vi "Graph_State_v00.vi"(4 "BS Hold Pulse":bool, 6 "\"I too high?\"":T6, 11 "Control Cavity Cluster":T11={"Control Pump A"={"Lock"=FALSE, "Hold"=FALSE, "P Gain"=0, "P BS"=-5, "I Gain"=0, "I BS"=-10, "I2 G"=0, "I2 BS"=-26, "Scan Amp"=0, "Scan Off"=0, "Scan FS"=0, "SFS BS"=0, "I Max value"=10000, "I2 Max value"=10000, "Scope.Offset"=0, "Trigger Direction"=enum."either", "Scan-PII thresh"=0}, "Control Pump B"={"Lock"=FALSE, "Hold"=FALSE, "P Gain"=0, "P BS"=-5, "I Gain"=0, "I BS"=-10, "I2 G"=0, "I2 BS"=-26, "Scan Amp"=0, "Scan Off"=0, "Scan FS"=0, "SFS BS"=0, "I Max value"=10000, "I2 Max value"=10000, "Scope.Offset"=0, "Trigger Direction"=enum."either", "Scan-PII thresh"=0}, "Control EPR"={"Lock"=FALSE, "Hold"=FALSE, "P Gain"=0, "P BS"=-5, "I Gain"=0, "I BS"=-10, "I2 G"=0, "I2 BS"=-26, "Scan Amp"=0, "Scan Off"=0, "Scan FS"=0, "SFS BS"=0, "I Max value"=10000, "I2 Max value"=10000, "Scope.Offset"=0, "Trigger Direction"=enum."either", "Scan-PII thresh"=0}, "Control Graph"={"Lock"=FALSE, "Hold"=FALSE, "P Gain"=0, "P BS"=-5, "I Gain"=0, "I BS"=-10, "I2 G"=0, "I2 BS"=-26, "Scan Amp"=0, "Scan Off"=0, "Scan FS"=0, "SFS BS"=0, "I Max value"=10000, "I2 Max value"=10000, "Scope.Offset"=0, "Trigger Direction"=enum."either", "Scan-PII thresh"=0}, "Control HD A"={"Lock"=FALSE, "Hold"=FALSE, "P Gain"=0, "P BS"=-5, "I Gain"=0, "I BS"=-10, "I2 G"=0, "I2 BS"=-26, "Scan Amp"=0, "Scan Off"=0, "Scan FS"=0, "SFS BS"=0, "I Max value"=10000, "I2 Max value"=10000, "Scope.Offset"=0, "Trigger Direction"=enum."either", "Scan-PII thresh"=0}, "Control HD B"={"Lock"=FALSE, "Hold"=FALSE, "P Gain"=0, "P BS"=-5, "I Gain"=0, "I BS"=-10, "I2 G"=0, "I2 BS"=-26, "Scan Amp"=0, "Scan Off"=0, "Scan FS"=0, "SFS BS"=0, "I Max value"=10000, "I2 Max value"=10000, "Scope.Offset"=0, "Trigger Direction"=enum."either", "Scan-PII thresh"=0}, "Max"={"Max Pump A"=0, "Max Pump B"=0, "Max EPR"=0, "Max Graph"=0, "Max HD A"=0, "Max HD B"=0}, "Min"={"Min Pump A"=0, "Min Pump B"=0, "Min EPR"=0, "Min Graph"=0, "Min HD A"=0, "Min HD B"=0}, "Lock Threshold"={"Pump A"=0, "Pump B"=0, "EPR"=0, "Graph"=0, "HD A"=0, "HD B"=0}, "Re-Scan Threshold"={"Pump A"=0, "Pump B"=0, "EPR"=0, "Graph"=0, "HD A"=40, "HD B"=0}, "Lock Point?"={"Pump A"=FALSE, "Pump B"=FALSE, "EPR"=FALSE, "Graph"=FALSE, "HD A"=FALSE, "HD B"=FALSE}, "Re-scan?"={"Pump A"=FALSE, "Pump B"=FALSE, "EPR"=FALSE, "Graph"=FALSE, "HD A"=FALSE, "HD B"=FALSE}, "Lock pressed? (-1)"={"Pump A"=FALSE, "Pump B"=FALSE, "EPR"=FALSE, "Graph"=FALSE, "HD A"=FALSE, "HD B"=FALSE}, "Cavity Errors"={"Pump A"=0, "Pump B"=0, "EPR"=0, "Graph"=0, "HD A"=0, "HD B"=0}, "State (-1)"={"Pump A"=enum."Safe", "Pump B"=enum."Safe", "EPR"=enum."Safe", "Graph"=enum."Safe", "HD A"=enum."Safe", "HD B"=enum."Safe"}, "Safety First"={"lim reset"=FALSE, "no limit"=FALSE, "pos slew rate * dt"=0, "neg slew rate * dt"=-5, "Hold All"=FALSE, "Count(Ticks)"=4294967286}}) -> (3 "PII Scan State Errors":T8={"Control Pump A"={"Lock"=FALSE, "Hold"=FALSE, "P Gain"=3, "P BS"=0, "I Gain"=0, "I BS"=-10, "I2 G"=0, "I2 BS"=-26, "Scan Amp"=0, "Scan Off"=0, "Scan FS"=0, "SFS BS"=0, "I Max value"=10000, "I2 Max value"=10000, "Scope.Offset"=0, "Trigger Direction"=enum."either", "Scan-PII thresh"=0}, "Control Pump B"={"Lock"=FALSE, "Hold"=FALSE, "P Gain"=0, "P BS"=-5, "I Gain"=0, "I BS"=-10, "I2 G"=0, "I2 BS"=-26, "Scan Amp"=0, "Scan Off"=0, "Scan FS"=0, "SFS BS"=0, "I Max value"=10000, "I2 Max value"=10000, "Scope.Offset"=0, "Trigger Direction"=enum."either", "Scan-PII thresh"=0}, "Control EPR"={"Lock"=FALSE, "Hold"=FALSE, "P Gain"=0, "P BS"=-5, "I Gain"=0, "I BS"=-10, "I2 G"=0, "I2 BS"=-26, "Scan Amp"=0, "Scan Off"=0, "Scan FS"=0, "SFS BS"=0, "I Max value"=10000, "I2 Max value"=10000, "Scope.Offset"=0, "Trigger Direction"=enum."either", "Scan-PII thresh"=0}, "Control Graph"={"Lock"=FALSE, "Hold"=FALSE, "P Gain"=0, "P BS"=-5, "I Gain"=0, "I BS"=-10, "I2 G"=0, "I2 BS"=-26, "Scan Amp"=0, "Scan Off"=0, "Scan FS"=0, "SFS BS"=0, "I Max value"=10000, "I2 Max value"=10000, "Scope.Offset"=0, "Trigger Direction"=enum."either", "Scan-PII thresh"=0}, "Control HD A"={"Lock"=FALSE, "Hold"=FALSE, "P Gain"=0, "P BS"=0, "I Gain"=0, "I BS"=-10, "I2 G"=0, "I2 BS"=-26, "Scan Amp"=0, "Scan Off"=0, "Scan FS"=0, "SFS BS"=0, "I Max value"=10000, "I2 Max value"=10000, "Scope.Offset"=0, "Trigger Direction"=enum."either", "Scan-PII thresh"=0}, "Control HD B"={"Lock"=FALSE, "Hold"=FALSE, "P Gain"=0, "P BS"=0, "I Gain"=0, "I BS"=-10, "I2 G"=0, "I2 BS"=-26, "Scan Amp"=0, "Scan Off"=0, "Scan FS"=0, "SFS BS"=0, "I Max value"=10000, "I2 Max value"=10000, "Scope.Offset"=0, "Trigger Direction"=enum."either", "Scan-PII thresh"=0}, "Error Signals"={"Pump A"=0, "Pump B"=0, "EPR"=0, "Graph"=0, "HD A"=0, "HD B"=0}, "State"={"Pump A"=enum."Safe", "Pump B"=enum."Safe", "EPR"=enum."Safe", "Graph"=enum."Safe", "HD A"=enum."Safe", "HD B"=enum."Safe"}}, 5 "MaxMin":T1)   [LabVIEW 2010]
doc: "The state of the output is decided here. There are four possible states: 1) Safe - zeros; 2) Hold - constant output of last value; 3) Scan - saw tooth at low frequency 4) Lock - PII output."
uses:
  Strict Type Defs/Graph State.ctl
  Strict Type Defs/Graph PII Scan State.ctl
  Strict Type Defs/PII individual.ctl
  Strict Type Defs/Graph Errors.ctl
  Strict Type Defs/Graph Lock Point.ctl
  Strict Type Defs/Graph Control Cluster.ctl
  Strict Type Defs/Graph Max.ctl
  Strict Type Defs/Graph Min.ctl
  Strict Type Defs/Lock Thresh Graph.ctl
  Strict Type Defs/Safety First.ctl
  Strict Type Defs/Graph MaxMin.ctl
  Strict Type Defs/Graph Reset MaxMin.ctl
panel:
  in  "MaxMin typedef":T1
  in  "Lock?":T6
  in  "PII Scan State":T8={"Control Pump A"={"Lock"=FALSE, "Hold"=FALSE, "P Gain"=3, "P BS"=0, "I Gain"=0, "I BS"=-10, "I2 G"=0, "I2 BS"=-26, "Scan Amp"=0, "Scan Off"=0, "Scan FS"=0, "SFS BS"=0, "I Max value"=10000, "I2 Max value"=10000, "Scope.Offset"=0, "Trigger Direction"=enum."either", "Scan-PII thresh"=0}, "Control Pump B"={"Lock"=FALSE, "Hold"=FALSE, "P Gain"=0, "P BS"=-5, "I Gain"=0, "I BS"=-10, "I2 G"=0, "I2 BS"=-26, "Scan Amp"=0, "Scan Off"=0, "Scan FS"=0, "SFS BS"=0, "I Max value"=10000, "I2 Max value"=10000, "Scope.Offset"=0, "Trigger Direction"=enum."either", "Scan-PII thresh"=0}, "Control EPR"={"Lock"=FALSE, "Hold"=FALSE, "P Gain"=0, "P BS"=-5, "I Gain"=0, "I BS"=-10, "I2 G"=0, "I2 BS"=-26, "Scan Amp"=0, "Scan Off"=0, "Scan FS"=0, "SFS BS"=0, "I Max value"=10000, "I2 Max value"=10000, "Scope.Offset"=0, "Trigger Direction"=enum."either", "Scan-PII thresh"=0}, "Control Graph"={"Lock"=FALSE, "Hold"=FALSE, "P Gain"=0, "P BS"=-5, "I Gain"=0, "I BS"=-10, "I2 G"=0, "I2 BS"=-26, "Scan Amp"=0, "Scan Off"=0, "Scan FS"=0, "SFS BS"=0, "I Max value"=10000, "I2 Max value"=10000, "Scope.Offset"=0, "Trigger Direction"=enum."either", "Scan-PII thresh"=0}, "Control HD A"={"Lock"=FALSE, "Hold"=FALSE, "P Gain"=0, "P BS"=0, "I Gain"=0, "I BS"=-10, "I2 G"=0, "I2 BS"=-26, "Scan Amp"=0, "Scan Off"=0, "Scan FS"=0, "SFS BS"=0, "I Max value"=10000, "I2 Max value"=10000, "Scope.Offset"=0, "Trigger Direction"=enum."either", "Scan-PII thresh"=0}, "Control HD B"={"Lock"=FALSE, "Hold"=FALSE, "P Gain"=0, "P BS"=0, "I Gain"=0, "I BS"=-10, "I2 G"=0, "I2 BS"=-26, "Scan Amp"=0, "Scan Off"=0, "Scan FS"=0, "SFS BS"=0, "I Max value"=10000, "I2 Max value"=10000, "Scope.Offset"=0, "Trigger Direction"=enum."either", "Scan-PII thresh"=0}, "Error Signals"={"Pump A"=0, "Pump B"=0, "EPR"=0, "Graph"=0, "HD A"=0, "HD B"=0}, "State"={"Pump A"=enum."Safe", "Pump B"=enum."Safe", "EPR"=enum."Safe", "Graph"=enum."Safe", "HD A"=enum."Safe", "HD B"=enum."Safe"}}
  in  "State":T2
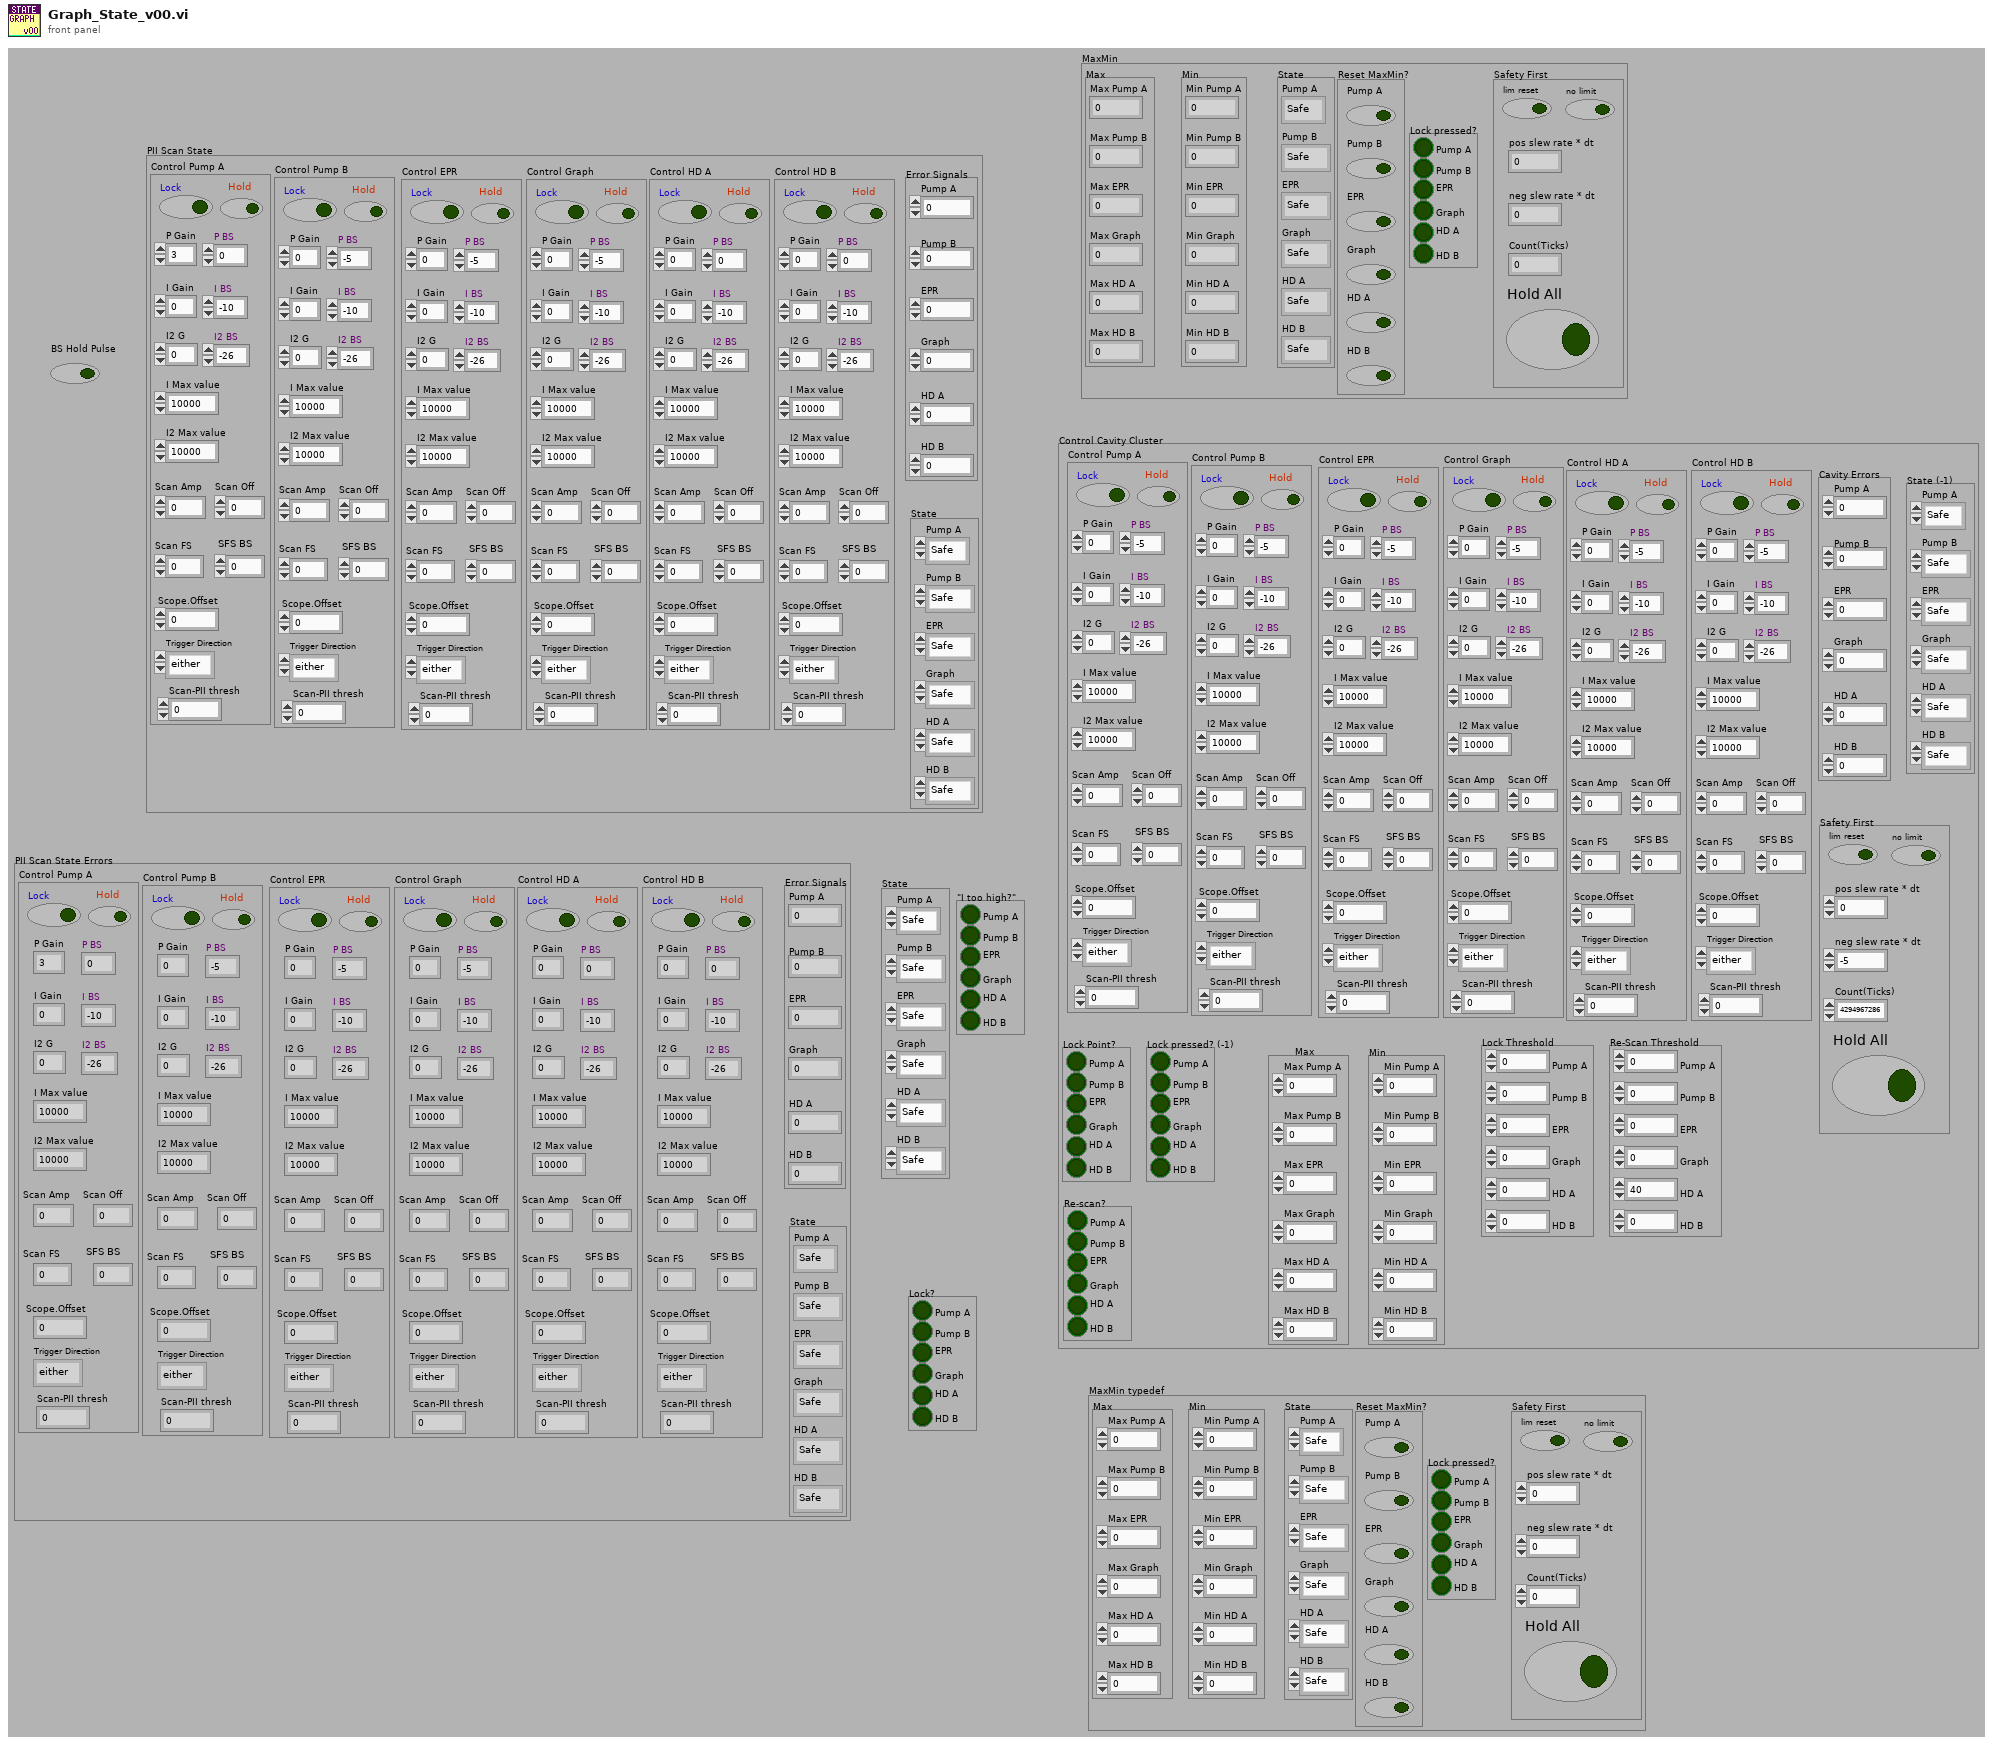
[diagram p1: front panel]
types:
  T1 = typedef "Graph MaxMin.ctl" = cluster{"State":T2, "Reset MaxMin?":T3, "Max":T4, "Min":T5, "Lock pressed?":T6, "Safety First":T7}
  T2 = typedef "Graph State.ctl" = cluster{"Pump A":enum16{"Safe", "Hold", "Scan", "Lock"}, "Pump B":enum16{"Safe", "Hold", "Scan", "Lock"}, "EPR":enum16{"Safe", "Hold", "Scan", "Lock"}, "Graph":enum16{"Safe", "Hold", "Scan", "Lock"}, "HD A":enum16{"Safe", "Hold", "Scan", "Lock"}, "HD B":enum16{"Safe", "Hold", "Scan", "Lock"}}
  T3 = typedef "Graph Reset MaxMin.ctl" = cluster{"Pump A":bool, "Pump B":bool, "EPR":bool, "Graph":bool, "HD A":bool, "HD B":bool}
  T4 = typedef "Graph Max.ctl" = cluster{"Max Pump A":i16, "Max Pump B":i16, "Max EPR":i16, "Max Graph":i16, "Max HD A":i16, "Max HD B":i16}
  T5 = typedef "Graph Min.ctl" = cluster{"Min Pump A":i16, "Min Pump B":i16, "Min EPR":i16, "Min Graph":i16, "Min HD A":i16, "Min HD B":i16}
  T6 = typedef "Graph Lock Point.ctl" = cluster{"Pump A":bool, "Pump B":bool, "EPR":bool, "Graph":bool, "HD A":bool, "HD B":bool}
  T7 = typedef "Safety First.ctl" = cluster{"lim reset":bool, "no limit":bool, "pos slew rate * dt":i16, "neg slew rate * dt":i16, "Hold All":bool, "Count(Ticks)":u32}
  T8 = typedef "Graph PII Scan State.ctl" = cluster{"Control Pump A":T9, "Control Pump B":T9, "Control EPR":T9, "Control Graph":T9, "Control HD A":T9, "Control HD B":T9, "Error Signals":T10, "State":T2}
  T9 = typedef "PII individual.ctl" = cluster{"Lock":bool, "Hold":bool, "P Gain":i32, "P BS":i16, "I Gain":i32, "I BS":i16, "I2 G":i32, "I2 BS":i16, "Scan Amp":i16, "Scan Off":i16, "Scan FS":u16, "SFS BS":i16, "I Max value":i32, "I2 Max value":i32, "Scope.Offset":i16, "Trigger Direction":enum8{"either", "minus-plus", "plus-minus"}, "Scan-PII thresh":i16}
  T10 = typedef "Graph Errors.ctl" = cluster{"Pump A":i16, "Pump B":i16, "EPR":i16, "Graph":i16, "HD A":i16, "HD B":i16}
  T11 = typedef "Graph Control Cluster.ctl" = cluster{"Control Pump A":T9, "Control Pump B":T9, "Control EPR":T9, "Control Graph":T9, "Control HD A":T9, "Control HD B":T9, "Max":T4, "Min":T5, "Lock Threshold":T12, "Re-Scan Threshold":T12, "Lock Point?":T6, "Re-scan?":T6, "Lock pressed? (-1)":T6, "Cavity Errors":T10, "State (-1)":T2, "Safety First":T7}
  T12 = typedef "Lock Thresh Graph.ctl" = cluster{"Pump A":i16, "Pump B":i16, "EPR":i16, "Graph":i16, "HD A":i16, "HD B":i16}
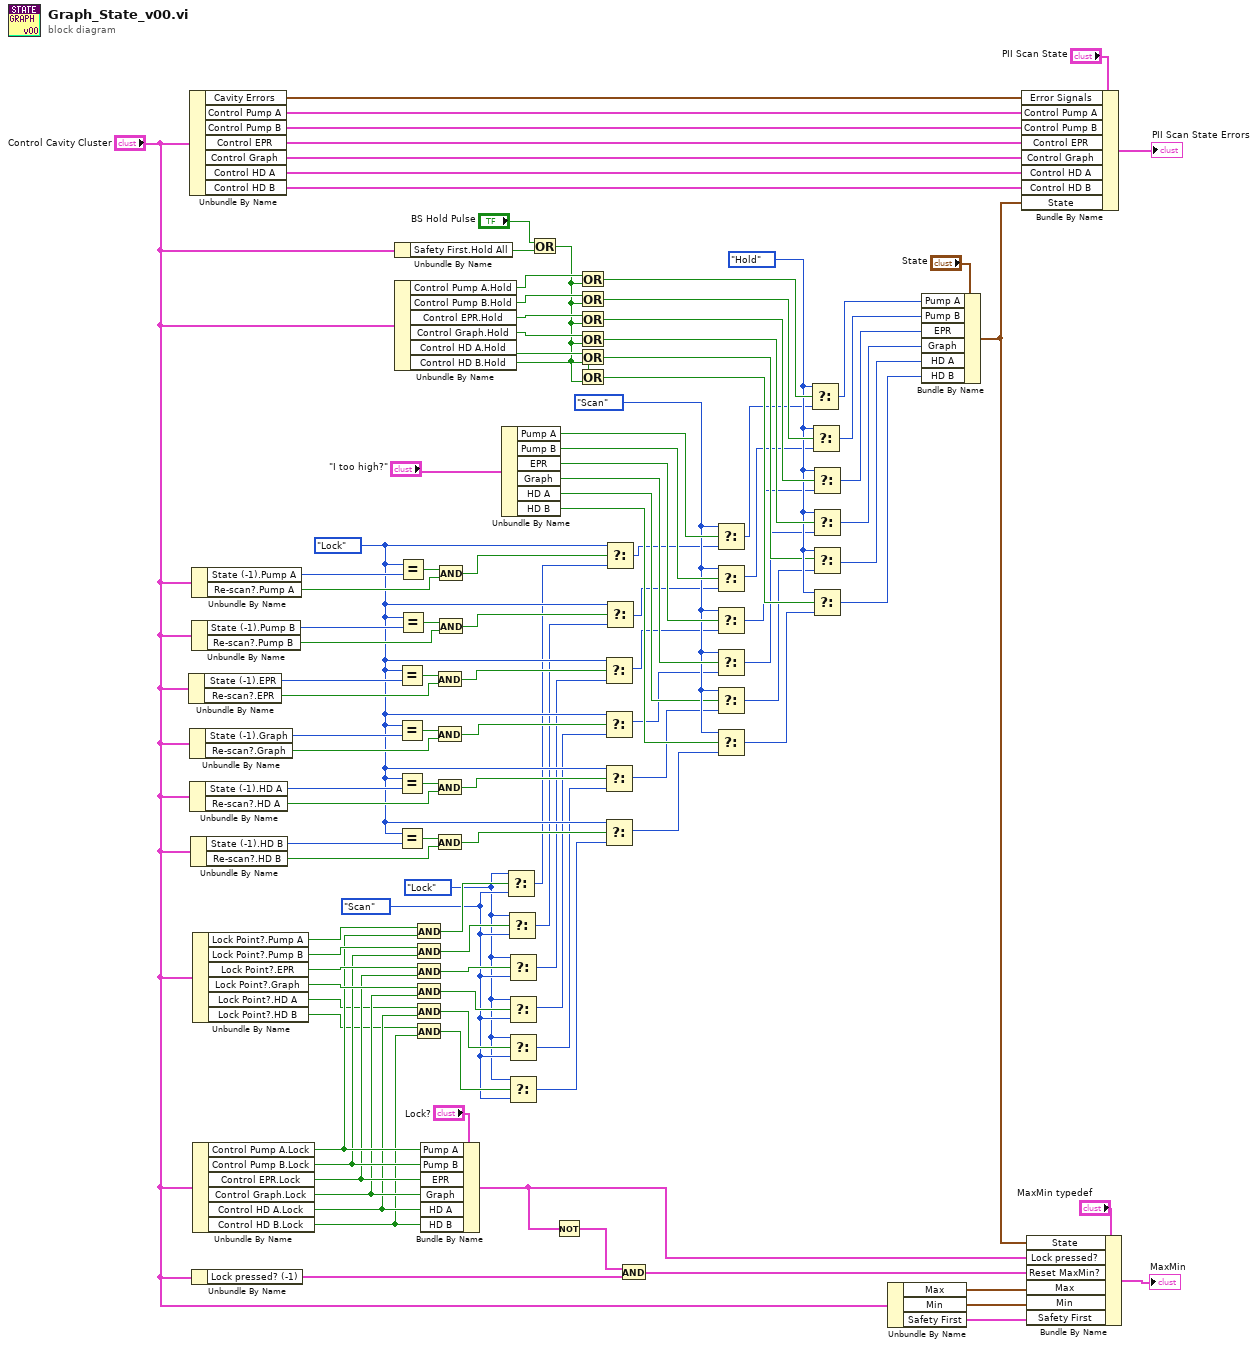
[diagram p0: block diagram]
diagram:
  w36 = enum16{"Safe", "Hold", "Scan", "Lock"}."Scan" ("State")
  w47 = enum16{"Safe", "Hold", "Scan", "Lock"}."Lock" ("y")
  w37 = enum16{"Safe", "Hold", "Scan", "Lock"}."Hold" ("State")
  w39 = enum16{"Safe", "Hold", "Scan", "Lock"}."Scan" ("State")
  w38 = enum16{"Safe", "Hold", "Scan", "Lock"}."Lock" ("State")
  n1 = Unbundle By Name("Control Cavity Cluster") -> ("State (-1).EPR"=w62:enum16{"Safe", "Hold", "Scan", "Lock"}, "Re-scan?.EPR"=w93:bool)
  n2 = Unbundle By Name("Control Cavity Cluster") -> ("Cavity Errors"=w89:T10, "Control Pump A"=w88:T9, "Control Pump B"=w87:T9, "Control EPR"=w86:T9, "Control Graph"=w85:T9, "Control HD A"=w45:T9, "Control HD B"=w44:T9)
  n3 = Unbundle By Name("Control Cavity Cluster") -> ("State (-1).Graph"=w63:enum16{"Safe", "Hold", "Scan", "Lock"}, "Re-scan?.Graph"=w94:bool)
  n4 = Unbundle By Name("Control Cavity Cluster") -> ("State (-1).HD A"=w55:enum16{"Safe", "Hold", "Scan", "Lock"}, "Re-scan?.HD A"=w51:bool)
  n5 = Unbundle By Name("Control Cavity Cluster") -> ("State (-1).HD B"=w54:enum16{"Safe", "Hold", "Scan", "Lock"}, "Re-scan?.HD B"=w50:bool)
  n6 = Unbundle By Name("Control Cavity Cluster") -> ("State (-1).Pump A"=w60:enum16{"Safe", "Hold", "Scan", "Lock"}, "Re-scan?.Pump A"=w100:bool)
  n7 = Unbundle By Name("Control Cavity Cluster") -> ("State (-1).Pump B"=w61:enum16{"Safe", "Hold", "Scan", "Lock"}, "Re-scan?.Pump B"=w99:bool)
  n8 = Unbundle By Name("Control Cavity Cluster") -> ("Lock pressed? (-1)"=w82:T6)
  n9 = Unbundle By Name("Control Cavity Cluster") -> ("Lock Point?.Pump A"=w71:bool, "Lock Point?.Pump B"=w70:bool, "Lock Point?.EPR"=w69:bool, "Lock Point?.Graph"=w68:bool, "Lock Point?.HD A"=w31:bool, "Lock Point?.HD B"=w29:bool)
  n10 = Unbundle By Name("Control Cavity Cluster") -> ("Control Pump A.Lock"=w67:bool, "Control Pump B.Lock"=w66:bool, "Control EPR.Lock"=w65:bool, "Control Graph.Lock"=w64:bool, "Control HD A.Lock"=w30:bool, "Control HD B.Lock"=w28:bool)
  n11 = Unbundle By Name("Control Cavity Cluster") -> ("Safety First.Hold All"=w15:bool)
  n12 = Unbundle By Name("Control Cavity Cluster") -> ("Control Pump A.Hold"=w107:bool, "Control Pump B.Hold"=w74:bool, "Control EPR.Hold"=w73:bool, "Control Graph.Hold"=w72:bool, "Control HD A.Hold"=w43:bool, "Control HD B.Hold"=w42:bool)
  n13 = Equal?(x=w47, y=w62) -> (x = y?=w92:bool)
  n14 = Equal?(x=w47, y=w63) -> (x = y?=w95:bool)
  n15 = Equal?(x=w47, y=w55) -> (x = y?=w52:bool)
  n16 = Equal?(x=w47, y=w54) -> (x = y?=w49:bool)
  n17 = Equal?(x=w47, y=w60) -> (x = y?=w101:bool)
  n18 = Equal?(x=w47, y=w61) -> (x = y?=w98:bool)
  n19 = And(x=w71, y=w67) -> (x .and. y?=w110:bool)
  n20 = And(x=w70, y=w66) -> (x .and. y?=w111:bool)
  n21 = And(x=w69, y=w65) -> (x .and. y?=w112:bool)
  n22 = And(x=w68, y=w64) -> (x .and. y?=w113:bool)
  n23 = And(x=w31, y=w30) -> (x .and. y?=w41:bool)
  n24 = And(x=w29, y=w28) -> (x .and. y?=w40:bool)
  n25 = Bundle By Name(cluster="Lock?", "Pump A"=w67, "Pump B"=w66, "EPR"=w65, "Graph"=w64, "HD A"=w30, "HD B"=w28) -> (w57:T6)
  n26 = And(x=w92, y=w93) -> (x .and. y?=w91:bool)
  n27 = And(x=w95, y=w94) -> (x .and. y?=w96:bool)
  n28 = And(x=w52, y=w51) -> (x .and. y?=w53:bool)
  n29 = And(x=w49, y=w50) -> (x .and. y?=w48:bool)
  n30 = And(x=w101, y=w100) -> (x .and. y?=w108:bool)
  n31 = And(x=w98, y=w99) -> (x .and. y?=w97:bool)
  n32 = Unbundle By Name("\"I too high?\"") -> ("Pump A"=w102:bool, "Pump B"=w78:bool, "EPR"=w77:bool, "Graph"=w76:bool, "HD A"=w33:bool, "HD B"=w32:bool)
  n33 = Select(t=w38, s=w110, f=w39) -> (s? t:f=w27:enum16{"Safe", "Hold", "Scan", "Lock"})
  n34 = Select(t=w38, s=w111, f=w39) -> (s? t:f=w26:enum16{"Safe", "Hold", "Scan", "Lock"})
  n35 = Select(t=w38, s=w112, f=w39) -> (s? t:f=w25:enum16{"Safe", "Hold", "Scan", "Lock"})
  n36 = Select(t=w38, s=w113, f=w39) -> (s? t:f=w24:enum16{"Safe", "Hold", "Scan", "Lock"})
  n37 = Select(t=w38, s=w41, f=w39) -> (s? t:f=w23:enum16{"Safe", "Hold", "Scan", "Lock"})
  n38 = Select(t=w38, s=w40, f=w39) -> (s? t:f=w22:enum16{"Safe", "Hold", "Scan", "Lock"})
  n39 = Or(x="BS Hold Pulse", y=w15) -> (x .or. y?=w13:bool)
  n40 = Not(x=w57) -> (.not. x?=w90:T6)
  n41 = Or(x=w107, y=w13) -> (x .or. y?=w106:bool)
  n42 = Or(x=w74, y=w13) -> (x .or. y?=w105:bool)
  n43 = Or(x=w73, y=w13) -> (x .or. y?=w104:bool)
  n44 = Or(x=w72, y=w13) -> (x .or. y?=w103:bool)
  n45 = Or(x=w43, y=w13) -> (x .or. y?=w35:bool)
  n46 = Or(x=w42, y=w13) -> (x .or. y?=w34:bool)
  n47 = Select(t=w47, s=w91, f=w25) -> (s? t:f=w19:enum16{"Safe", "Hold", "Scan", "Lock"})
  n48 = Select(t=w47, s=w96, f=w24) -> (s? t:f=w18:enum16{"Safe", "Hold", "Scan", "Lock"})
  n49 = Select(t=w47, s=w53, f=w23) -> (s? t:f=w17:enum16{"Safe", "Hold", "Scan", "Lock"})
  n50 = Select(t=w47, s=w48, f=w22) -> (s? t:f=w16:enum16{"Safe", "Hold", "Scan", "Lock"})
  n51 = Select(t=w47, s=w108, f=w27) -> (s? t:f=w21:enum16{"Safe", "Hold", "Scan", "Lock"})
  n52 = Select(t=w47, s=w97, f=w26) -> (s? t:f=w20:enum16{"Safe", "Hold", "Scan", "Lock"})
  n53 = And(x=w90, y=w82) -> (x .and. y?=w80:T6)
  n54 = Select(t=w36, s=w102, f=w21) -> (s? t:f=w12:enum16{"Safe", "Hold", "Scan", "Lock"})
  n55 = Select(t=w36, s=w78, f=w20) -> (s? t:f=w11:enum16{"Safe", "Hold", "Scan", "Lock"})
  n56 = Select(t=w36, s=w77, f=w19) -> (s? t:f=w10:enum16{"Safe", "Hold", "Scan", "Lock"})
  n57 = Select(t=w36, s=w76, f=w18) -> (s? t:f=w9:enum16{"Safe", "Hold", "Scan", "Lock"})
  n58 = Select(t=w36, s=w33, f=w17) -> (s? t:f=w8:enum16{"Safe", "Hold", "Scan", "Lock"})
  n59 = Select(t=w36, s=w32, f=w16) -> (s? t:f=w7:enum16{"Safe", "Hold", "Scan", "Lock"})
  n60 = Select(t=w37, s=w106, f=w12) -> (s? t:f=w6:enum16{"Safe", "Hold", "Scan", "Lock"})
  n61 = Select(t=w37, s=w105, f=w11) -> (s? t:f=w5:enum16{"Safe", "Hold", "Scan", "Lock"})
  n62 = Select(t=w37, s=w104, f=w10) -> (s? t:f=w4:enum16{"Safe", "Hold", "Scan", "Lock"})
  n63 = Select(t=w37, s=w103, f=w9) -> (s? t:f=w3:enum16{"Safe", "Hold", "Scan", "Lock"})
  n64 = Select(t=w37, s=w35, f=w8) -> (s? t:f=w2:enum16{"Safe", "Hold", "Scan", "Lock"})
  n65 = Select(t=w37, s=w34, f=w7) -> (s? t:f=w1:enum16{"Safe", "Hold", "Scan", "Lock"})
  n66 = Unbundle By Name("Control Cavity Cluster") -> ("Max"=w59:T4, "Min"=w58:T5, "Safety First"=w56:T7)
  n67 = Bundle By Name(cluster="State", "Pump A"=w6, "Pump B"=w5, "EPR"=w4, "Graph"=w3, "HD A"=w2, "HD B"=w1) -> (w79:T2)
  n68 = Bundle By Name(cluster="PII Scan State", "Error Signals"=w89, "Control Pump A"=w88, "Control Pump B"=w87, "Control EPR"=w86, "Control Graph"=w85, "Control HD A"=w45, "Control HD B"=w44, "State"=w79) -> (→"PII Scan State Errors":T8)
  n69 = Bundle By Name(cluster="MaxMin typedef", "State"=w79, "Lock pressed?"=w57, "Reset MaxMin?"=w80, "Max"=w59, "Min"=w58, "Safety First"=w56) -> (→"MaxMin":T1)
